vi "libssh2_channel_direct_tcpip_ex.vi"(4 "sport":i32, 6 "shost":string, 8 "error in (no error)":errorcluster, 9 "port":i32, 10 "host":string, 11 "session":u64) -> (0 "error out":errorcluster, 3 "return value":u64)   [LabVIEW 2013, in "libssh2.lvlib"]
uses:
  libssh2.lvlib
  libssh2.dll
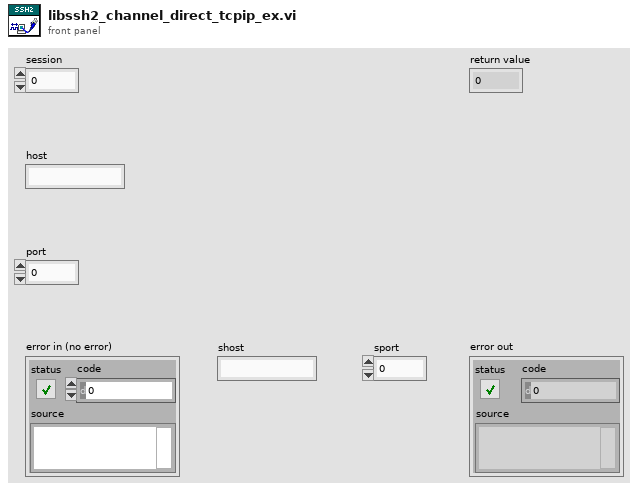
[diagram p1: front panel]
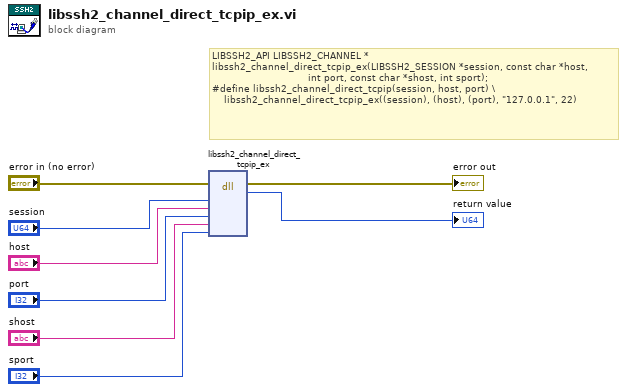
[diagram p0: block diagram]
diagram:
  # "LIBSSH2_API LIBSSH2_CHANNEL *\nlibssh2_channel_direct_tcpip_ex(LIBSSH2_SESSION *session, const char *host,\n                                int port, const char *shost, int sport);\n#define libssh2_channel_direct_tcpip(session, host, port) \\\n    libssh2_channel_direct_tcpip_ex((session), (host), (port), \"127.0.0.1\", 22)"
  n1 = dll-call lib="C:/Users/pasca/source/repos/libssh2-labview/libssh2**.*" fn="libssh2_channel_direct_tcpip_ex"(error in="error in (no error)", "session"="session", "host"="host", "port"="port", "shost"="shost", "sport"="sport") -> (error out=→"error out":errorcluster, "return value"=→"return value":u64)  [unwired: 7 in, 1 out]
